vi "STS_IterableDAQ_BK2841.vi"() -> ()   [LabVIEW 2021]
uses:
  <vilib>/express/express analysis/Spectral/Block/exnSpectralBlock spectral measurements RMS poly.vi
  <vilib>/express/express analysis/Spectral/Block/exnSpectralBlock spectral measurements RMS DDT.vi
  <vilib>/express/express analysis/Spectral/XNode/ExpressSpectralMeasurementsBlockNode.xnode
  <vilib>/regexp/Match Regular Expression.xnode
panel:
  in  "Tab Control":enum32{"Page 1", "Page 2"}(tab)
  out "Up Light":bool
  out "Down Light":bool
  out "Acceleration":dynamicdata(graph)
  out "FFT":dynamicdata(graph) caption="Fast Fourier Transform"
  in  "VISA resource name":refnum<visa-resource-name>
  out "BK Measurement":string
  out "Filename Out":path
  in  "Iterations?":i32
  out "Current Iteration":i32
  out "Numeric":dbl
  out "read buffer":string
  out "Resistance":dbl format="%#_6p"
  out "Temp":dbl
  out "Samples / Second":dbl
  out "Resistance Vs Time":dbl(graph)
  in  "Measurement mode":T1(ring)=enum."Resistance and Temp"
  in  "Display State":enum16{"Display ON", "Display OFF"}(ring)=enum."Display OFF"
  in  "Resistance measurement range":T2(ring)
  in  "measurement time":enum16{"FAST", "MED", "SLOW1", "SLOW2"}(ring)
  in  "Measurement speed":enum16{"FAST", "SLOW"}(ring)
  in  "measurement delay time (default 0.003)":dbl=0.003
  out "Array":dbl[](array[numeric])
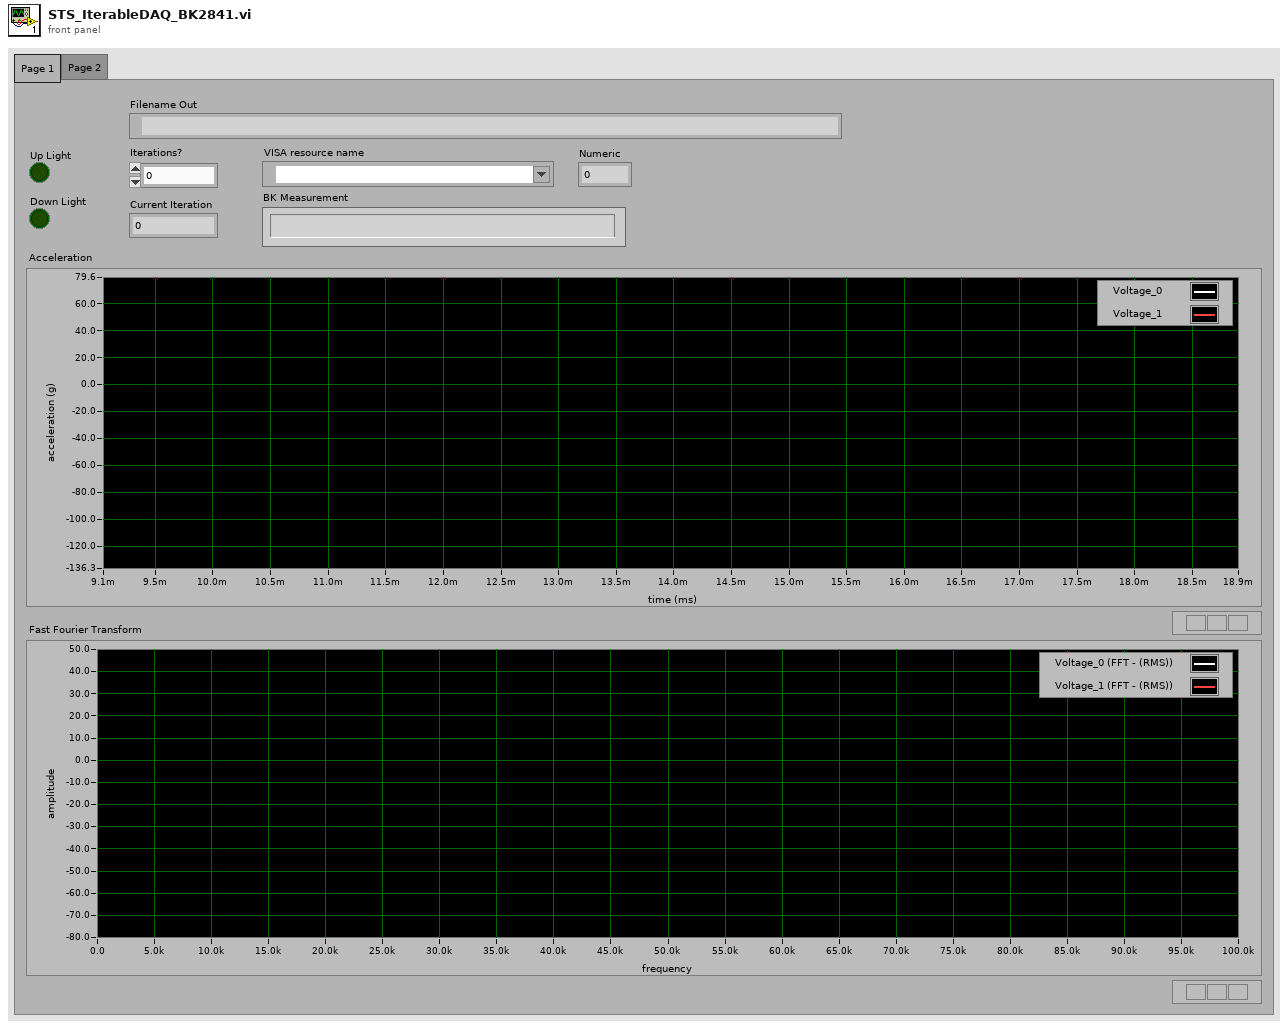
[diagram p1: front panel]
types:
  T1 = enum16{"Resistance", "Resistance and Temp", "Low Power Resistance", "Low Power Resisance and Temp", "Temp"}
  T2 = enum16{"Auto", "20 milli-Ohms", "200 milli-Ohms", "2 Ohms", "20 Ohms", "200 Ohms", "2 k-Ohms", "20 k-Ohms", "100 k-Ohms", "1 M-Ohms", "10 M-Ohms", "100 M-Ohms"}
  T3 = cluster{"averaging mode":u16, "weighting mode":u16, "number of averages":u32}
  T4 = cluster{"dB On (F)":bool, "unwrap phase (F)":bool, "convert to degree (F)":bool}
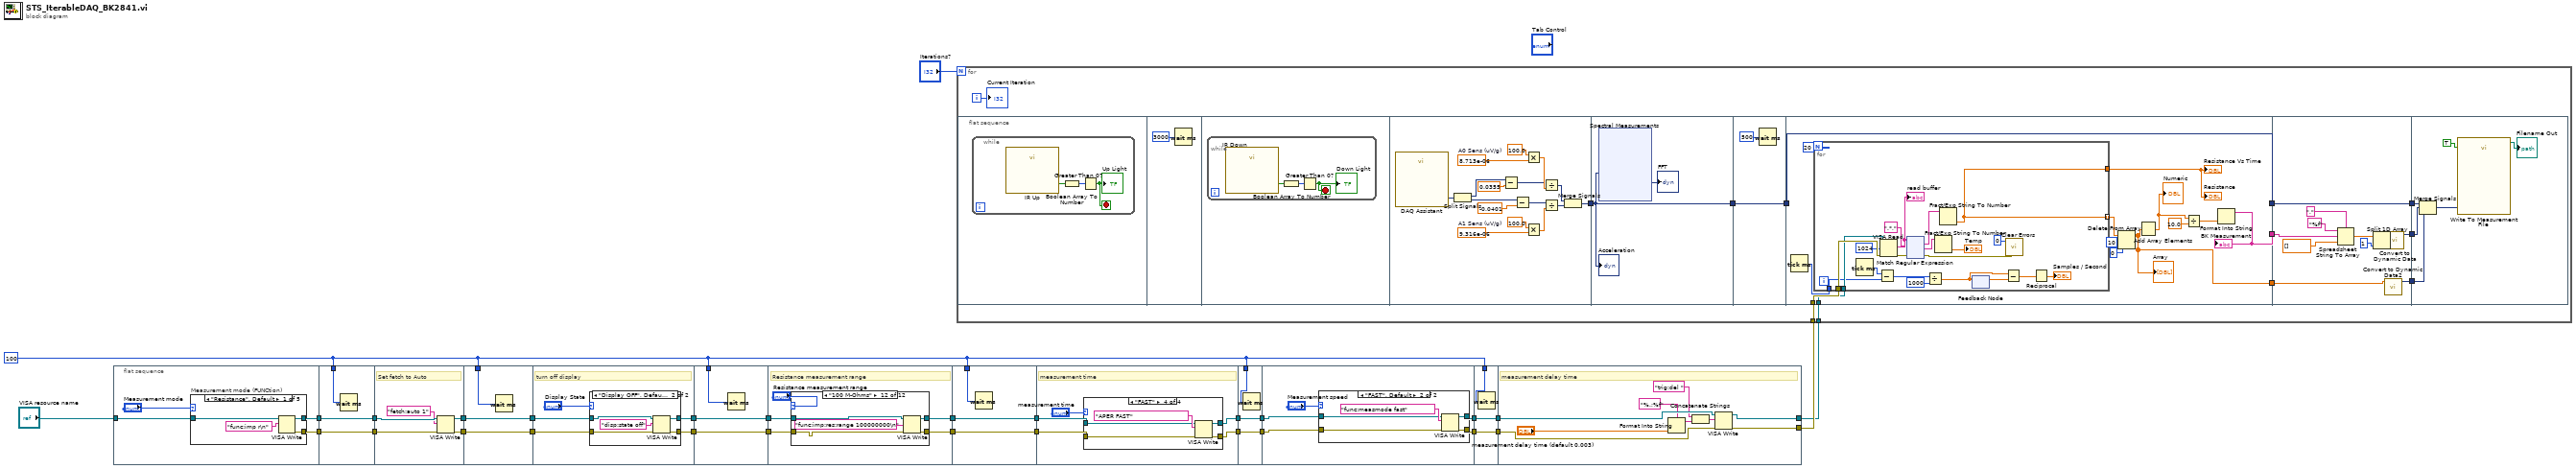
[diagram p0: block diagram]
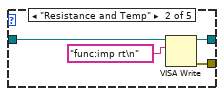
[diagram p2: hidden frame]
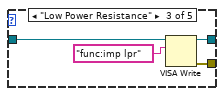
[diagram p3: hidden frame]
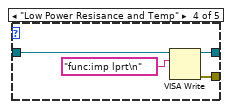
[diagram p4: hidden frame]
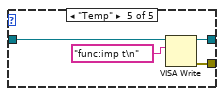
[diagram p5: hidden frame]
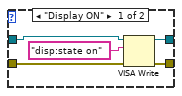
[diagram p6: hidden frame]
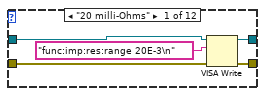
[diagram p7: hidden frame]
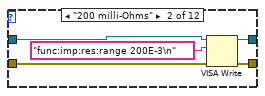
[diagram p8: hidden frame]
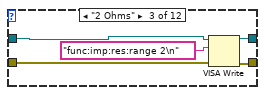
[diagram p9: hidden frame]
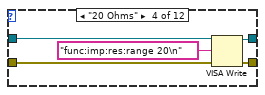
[diagram p10: hidden frame]
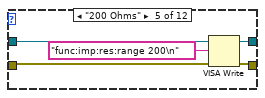
[diagram p11: hidden frame]
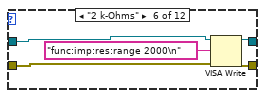
[diagram p12: hidden frame]
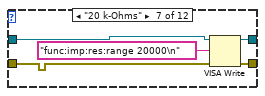
[diagram p13: hidden frame]
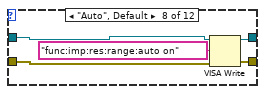
[diagram p14: hidden frame]
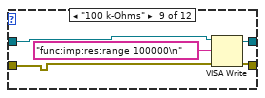
[diagram p15: hidden frame]
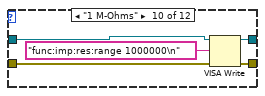
[diagram p16: hidden frame]
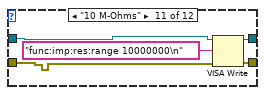
[diagram p17: hidden frame]
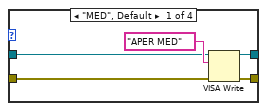
[diagram p18: hidden frame]
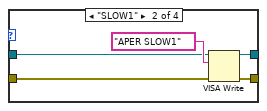
[diagram p19: hidden frame]
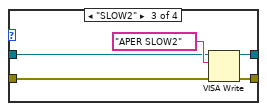
[diagram p20: hidden frame]
diagram:
  w4 = u32 100 ("delay before read (ms)")
  n1 = flat-sequence {
    tunnel: "VISA resource name" -> [w32]
    tunnel: [w30] -> w28
    tunnel: [w31] -> w27
    tunnel: [w56] -> w26
    tunnel: [w55] -> w25
    tunnel: w28 -> [w56]
    tunnel: w27 -> [w55]
    tunnel: w4 -> [w54]
    tunnel: w26 -> [w61]
    tunnel: w25 -> [w60]
    tunnel: [w59] -> w24
    tunnel: [w58] -> w23
    tunnel: w24 -> [w64]
    tunnel: w23 -> [w63]
    tunnel: w4 -> [w62]
    tunnel: [w64] -> w22
    tunnel: [w63] -> w21
    tunnel: w22 -> [w66]
    tunnel: w21 -> [w69]
    tunnel: [w68] -> w20
    tunnel: [w67] -> w19
    tunnel: w20 -> [w81]
    tunnel: w4 -> [w80]
    tunnel: w19 -> [w82]
    tunnel: [w82] -> w18
    tunnel: [w81] -> w17
    tunnel: w18 -> [w85]
    tunnel: w17 -> [w86]
    tunnel: [w83] -> w16
    tunnel: [w84] -> w15
    tunnel: w16 -> [w150]
    tunnel: w15 -> [w149]
    tunnel: [w150] -> w14
    tunnel: [w149] -> w13
    tunnel: w4 -> [w148]
    tunnel: w14 -> [w153]
    tunnel: w13 -> [w154]
    tunnel: [w151] -> w12
    tunnel: [w152] -> w11
    tunnel: w12 -> [w178]
    tunnel: w11 -> [w177]
    tunnel: [w178] -> w10
    tunnel: [w177] -> w9
    tunnel: w4 -> [w176]
    tunnel: w10 -> [w181]
    tunnel: w9 -> [w182]
    tunnel: [w180] -> w8
    tunnel: [w179] -> w7
    tunnel: w8 -> [w196]
    tunnel: w7 -> [w195]
    tunnel: [w196] -> w6
    tunnel: [w195] -> w5
    tunnel: w4 -> [w194]
    tunnel: [w202] -> w1
    tunnel: [w203] -> w2
    tunnel: w6 -> [w204]
    tunnel: w5 -> [w205]
    frame #0 {
      n2 = case "Measurement mode (FUNCtion)" shown="\"Resistance\", Default" "Measurement mode" {
        tunnel: w32 -> [w36 w41 w44 w48 w52]
        tunnel: [w35 w39 w43 w47 w51] -> w31
        tunnel: [w34 w38 w42 w46 w50] -> w30
        frame "Resistance", Default {
          n3 = VISA Write(VISA resource name=w36, write buffer="func:imp r\n") -> (VISA resource name out=w35:refnum<visa-resource-name>, error out=w34:errorcluster)  [unwired: 1 in, 1 out]
        }
        frame "Resistance and Temp" {
          n4 = VISA Write(VISA resource name=w41, write buffer="func:imp rt\n") -> (VISA resource name out=w39:refnum<visa-resource-name>, error out=w38:errorcluster)  [unwired: 1 in, 1 out]
        }
        frame "Low Power Resistance" {
          n5 = VISA Write(VISA resource name=w44, write buffer="func:imp lpr") -> (VISA resource name out=w43:refnum<visa-resource-name>, error out=w42:errorcluster)  [unwired: 1 in, 1 out]
        }
        frame "Low Power Resisance and Temp" {
          n6 = VISA Write(VISA resource name=w48, write buffer="func:imp lprt\n") -> (VISA resource name out=w47:refnum<visa-resource-name>, error out=w46:errorcluster)  [unwired: 1 in, 1 out]
        }
        frame "Temp" {
          n7 = VISA Write(VISA resource name=w52, write buffer="func:imp t\n") -> (VISA resource name out=w51:refnum<visa-resource-name>, error out=w50:errorcluster)  [unwired: 1 in, 1 out]
        }
      }
    }
    frame #1 {
      n8 = Wait (ms)(milliseconds to wait=w54) -> ()  [unwired: 1 out]
    }
    frame #2 {
      # "Set fetch to Auto"
      n9 = VISA Write(VISA resource name=w60, write buffer="fetch:auto 1", error in (no error)=w61) -> (VISA resource name out=w58:refnum<visa-resource-name>, error out=w59:errorcluster)  [unwired: 1 out]
    }
    frame #3 {
      n10 = Wait (ms)(milliseconds to wait=w62) -> ()  [unwired: 1 out]
    }
    frame #4 {
      # "turn off display"
      n11 = case shown="\"Display OFF\", Default" "Display State" {
        tunnel: w69 -> [w70 w78]
        tunnel: [w71 w77] -> w68
        tunnel: [w72 w76] -> w67
        tunnel: w66 -> [w73 w75]
        frame "Display ON" {
          n12 = VISA Write(VISA resource name=w70, write buffer="disp:state on", error in (no error)=w73) -> (VISA resource name out=w71:refnum<visa-resource-name>, error out=w72:errorcluster)  [unwired: 1 out]
        }
        frame "Display OFF", Default {
          n13 = VISA Write(VISA resource name=w78, write buffer="disp:state off", error in (no error)=w75) -> (VISA resource name out=w77:refnum<visa-resource-name>, error out=w76:errorcluster)  [unwired: 1 out]
        }
      }
    }
    frame #5 {
      n14 = Wait (ms)(milliseconds to wait=w80) -> ()  [unwired: 1 out]
    }
    frame #6 {
      # "Resistance measurement range"
      n15 = case shown="\"100 M-Ohms\"" "Resistance measurement range" {
        tunnel: w86 -> [w88 w96 w101 w104 w111 w113 w118 w123 w130 w133 w138 w144]
        tunnel: [w89 w95 w98 w106 w109 w116 w121 w126 w128 w136 w141 w146] -> w84
        tunnel: [w90 w94 w99 w105 w108 w115 w120 w125 w131 w135 w140 w145] -> w83
        tunnel: w85 -> [w91 w93 w100 w103 w110 w114 w119 w124 w129 w134 w139 w143]
        frame "20 milli-Ohms" {
          n16 = VISA Write(VISA resource name=w88, write buffer="func:imp:res:range 20E-3\n", error in (no error)=w91) -> (VISA resource name out=w89:refnum<visa-resource-name>, error out=w90:errorcluster)  [unwired: 1 out]
        }
        frame "200 milli-Ohms" {
          n17 = VISA Write(VISA resource name=w96, write buffer="func:imp:res:range 200E-3\n", error in (no error)=w93) -> (VISA resource name out=w95:refnum<visa-resource-name>, error out=w94:errorcluster)  [unwired: 1 out]
        }
        frame "2 Ohms" {
          n18 = VISA Write(VISA resource name=w101, write buffer="func:imp:res:range 2\n", error in (no error)=w100) -> (VISA resource name out=w98:refnum<visa-resource-name>, error out=w99:errorcluster)  [unwired: 1 out]
        }
        frame "20 Ohms" {
          n19 = VISA Write(VISA resource name=w104, write buffer="func:imp:res:range 20\n", error in (no error)=w103) -> (VISA resource name out=w106:refnum<visa-resource-name>, error out=w105:errorcluster)  [unwired: 1 out]
        }
        frame "200 Ohms" {
          n20 = VISA Write(VISA resource name=w111, write buffer="func:imp:res:range 200\n", error in (no error)=w110) -> (VISA resource name out=w109:refnum<visa-resource-name>, error out=w108:errorcluster)  [unwired: 1 out]
        }
        frame "2 k-Ohms" {
          n21 = VISA Write(VISA resource name=w113, write buffer="func:imp:res:range 2000\n", error in (no error)=w114) -> (VISA resource name out=w116:refnum<visa-resource-name>, error out=w115:errorcluster)  [unwired: 1 out]
        }
        frame "20 k-Ohms" {
          n22 = VISA Write(VISA resource name=w118, write buffer="func:imp:res:range 20000\n", error in (no error)=w119) -> (VISA resource name out=w121:refnum<visa-resource-name>, error out=w120:errorcluster)  [unwired: 1 out]
        }
        frame "Auto", Default {
          n23 = VISA Write(VISA resource name=w123, write buffer="func:imp:res:range:auto on", error in (no error)=w124) -> (VISA resource name out=w126:refnum<visa-resource-name>, error out=w125:errorcluster)  [unwired: 1 out]
        }
        frame "100 k-Ohms" {
          n24 = VISA Write(VISA resource name=w130, write buffer="func:imp:res:range 100000\n", error in (no error)=w129) -> (VISA resource name out=w128:refnum<visa-resource-name>, error out=w131:errorcluster)  [unwired: 1 out]
        }
        frame "1 M-Ohms" {
          n25 = VISA Write(VISA resource name=w133, write buffer="func:imp:res:range 1000000\n", error in (no error)=w134) -> (VISA resource name out=w136:refnum<visa-resource-name>, error out=w135:errorcluster)  [unwired: 1 out]
        }
        frame "10 M-Ohms" {
          n26 = VISA Write(VISA resource name=w138, write buffer="func:imp:res:range 10000000\n", error in (no error)=w139) -> (VISA resource name out=w141:refnum<visa-resource-name>, error out=w140:errorcluster)  [unwired: 1 out]
        }
        frame "100 M-Ohms" {
          n27 = VISA Write(VISA resource name=w144, write buffer="func:imp:res:range 100000000\n", error in (no error)=w143) -> (VISA resource name out=w146:refnum<visa-resource-name>, error out=w145:errorcluster)  [unwired: 1 out]
        }
      }
    }
    frame #7 {
      n28 = Wait (ms)(milliseconds to wait=w148) -> ()  [unwired: 1 out]
    }
    frame #8 {
      # "measurement time"
      n29 = case shown="\"FAST\"" "measurement time" {
        tunnel: w154 -> [w156 w164 w169 w171]
        tunnel: [w157 w163 w166 w174] -> w152
        tunnel: [w158 w162 w167 w173] -> w151
        tunnel: w153 -> [w159 w161 w168 w172]
        frame "MED", Default {
          n30 = VISA Write(VISA resource name=w156, write buffer="APER MED", error in (no error)=w159) -> (VISA resource name out=w157:refnum<visa-resource-name>, error out=w158:errorcluster)  [unwired: 1 out]
        }
        frame "SLOW1" {
          n31 = VISA Write(VISA resource name=w164, write buffer="APER SLOW1", error in (no error)=w161) -> (VISA resource name out=w163:refnum<visa-resource-name>, error out=w162:errorcluster)  [unwired: 1 out]
        }
        frame "SLOW2" {
          n32 = VISA Write(VISA resource name=w169, write buffer="APER SLOW2", error in (no error)=w168) -> (VISA resource name out=w166:refnum<visa-resource-name>, error out=w167:errorcluster)  [unwired: 1 out]
        }
        frame "FAST" {
          n33 = VISA Write(VISA resource name=w171, write buffer="APER FAST", error in (no error)=w172) -> (VISA resource name out=w174:refnum<visa-resource-name>, error out=w173:errorcluster)  [unwired: 1 out]
        }
      }
    }
    frame #9 {
      n34 = Wait (ms)(milliseconds to wait=w176) -> ()  [unwired: 1 out]
    }
    frame #10 {
      n35 = case shown="\"FAST\", Default" "Measurement speed" {
        tunnel: w182 -> [w187 w189]
        tunnel: [w186 w192] -> w179
        tunnel: [w185 w191] -> w180
        tunnel: w181 -> [w184 w190]
        frame "SLOW" {
          n36 = VISA Write(VISA resource name=w187, write buffer="func:measmode slow", error in (no error)=w184) -> (VISA resource name out=w186:refnum<visa-resource-name>, error out=w185:errorcluster)  [unwired: 1 out]
        }
        frame "FAST", Default {
          n37 = VISA Write(VISA resource name=w189, write buffer="func:measmode fast", error in (no error)=w190) -> (VISA resource name out=w192:refnum<visa-resource-name>, error out=w191:errorcluster)  [unwired: 1 out]
        }
      }
    }
    frame #11 {
      n38 = Wait (ms)(milliseconds to wait=w194) -> ()  [unwired: 1 out]
    }
    frame #12 {
      # "measurement delay time"
      n39 = Format Into String(format string="%.;%f", "measurement delay time (default 0.003)") -> (resulting string=w198:string)  [unwired: 2 in, 1 out]
      n40 = Concatenate Strings("trig:del " ("write buffer"), w198) -> (w197:string)
      n41 = VISA Write(VISA resource name=w205, write buffer=w197, error in (no error)=w204) -> (VISA resource name out=w202:refnum<visa-resource-name>, error out=w203:errorcluster)  [unwired: 1 out]
    }
  }
  n42 = for {
    N: "Iterations?" -> [_]
    tunnel: w2 -> [w209]
    tunnel: w1 -> [w208]
    i -> [w210]
    n43 = flat-sequence {
      tunnel: [w238] -> w217
      tunnel: w217 -> [w241]
      tunnel: [w241] -> w216
      tunnel: w216 -> [w253]
      tunnel: [w253] -> w215
      tunnel: [w265] -> w214
      tunnel: w215 -> [w268]
      tunnel: [w268] -> w213
      tunnel: w209 -> [w267]
      tunnel: w208 -> [w266]
      tunnel: [w255] -> w206
      tunnel: w214 -> [w408]
      tunnel: w213 -> [w409]
      tunnel: [w410] -> w212
      tunnel: [w409] -> w211
      tunnel: [w407] -> w207
      tunnel: w206 -> [w406]
      tunnel: w212 -> [w421]
      tunnel: w211 -> [w422]
      tunnel: w207 -> [w417]
      frame #0 {
        n44 = while {
          stop <- w219 stop-if-true
          n45 = call "IR Up"() -> ("data"=w218:bool[])  [unwired: 17 in, 2 out]
          n46 = Boolean Array To Number(Boolean array=w218) -> (number=w220:u32)
          n47 = Greater Than 0?(x=w220) -> (x > 0?=w219:bool)
          "Up Light" <- w219
        }
      }
      frame #1 {
        n48 = Wait (ms)(milliseconds to wait=u32 3000) -> ()  [unwired: 1 out]
      }
      frame #2 {
        n49 = while {
          stop <- w223 stop-if-true
          n50 = call "IR Down"() -> ("data"=w222:bool[])  [unwired: 17 in, 2 out]
          n51 = Boolean Array To Number(Boolean array=w222) -> (number=w224:u32)
          n52 = Greater Than 0?(x=w224) -> (x > 0?=w223:bool)
          "Down Light" <- w223
        }
      }
      frame #3 {
        w232 = 8.713e-06  # A0 Sens (uV/g)
        w228 = 9.316e-06  # A1 Sens (uV/g)
        n53 = call "DAQ Assistant"() -> ("data"=w237:dynamicdata)  [unwired: 17 in, 2 out]
        n54 = Split Signals(w237) -> (w235:dynamicdata, w236:dynamicdata)  [unwired: 2 in]
        n55 = Subtract(x=w235, y=0.0355) -> (x-y=w230:dynamicdata)
        n56 = Subtract(x=w236, y=-0.0401) -> (x-y=w226:dynamicdata)
        n57 = Multiply(x=100.0, y=w232) -> (x*y=w231:dbl)
        n58 = Multiply(x=100.0, y=w228) -> (x*y=w227:dbl)
        n59 = Divide(x=w230, y=w231) -> (x/y=w229:dynamicdata)
        n60 = Divide(x=w226, y=w227) -> (x/y=w225:dynamicdata)
        n61 = Merge Signals(w229, w225) -> (w238:dynamicdata)
      }
      frame #4 {
        n62 = xnode "Spectral Measurements"("Signals"=w241) -> ("FFT - (RMS)"=→"FFT":dynamicdata)  [unwired: 1 in, 2 out]
        "Acceleration" <- w241
      }
      frame #5 {
        n63 = Wait (ms)(milliseconds to wait=u32 500 ("delay before read (ms)")) -> ()  [unwired: 1 out]
      }
      frame #6 {
        n64 = Tick Count (ms)() -> (millisecond timer value=w264:u32)
        n65 = for {
          N: 20 -> [_]
          tunnel: w267 -> [w275]
          tunnel: w266 -> [w273]
          tunnel: w264 -> [w272]
          tunnel: [w271] -> w260
          tunnel: [w271] -> w258 mode=indexing
          n66 = Tick Count (ms)() -> (millisecond timer value=w282:u32)
          n67 = Subtract(x=w282, y=w272) -> (x-y=w284:u32)
          n68 = VISA Read(VISA resource name=w273, byte count=u32 1024, error in (no error)=w275) -> (read buffer=w281:string, error out=w280:errorcluster)  [unwired: 2 out]
          "read buffer" <- w281
          n69 = xnode "Match Regular Expression"("input string"=w281, "regular expression"=".*,", "error in"=w280) -> ("whole match"=w278:string, "after match"=w279:string, "error out"=w270:errorcluster)  [unwired: 3 in, 2 out]
          n70 = Divide(x=w284, y=u32 1000) -> (x/y=w285:dbl)
          n71 = Fract/Exp String To Number(string=w279) -> (number=→"Temp":dbl)  [unwired: 3 in, 1 out]
          n72 = Fract/Exp String To Number(string=w278) -> (number=w271:dbl)  [unwired: 3 in, 1 out]
          n73 = feedback #1() -> (w286:dbl)  [unwired: 1 in]
          n74 = feedback-in #1(w285) -> ()
          n75 = Subtract(x=w285, y=w286) -> (x-y=w287:dbl)
          n76 = call <vilib>:"Clear Errors.vi"("error in (no error)"=w270, "specific error code to clear (0: all)"=0) -> ()  [unwired: 4 in, 2 out]
          n77 = Reciprocal(x=w287) -> (1/x=→"Samples / Second":dbl)
        }
        "Resistance" <- w260
        "Resistance Vs Time" <- w260
        n78 = Delete From Array(array=w258, length=10, index=0) -> (array with subset deleted=w255:dbl[])  [unwired: 1 out]
        "Array" <- w255
        n79 = Add Array Elements(numeric array=w255) -> (sum=w259:dbl)
        "Numeric" <- w259
        n80 = Divide(x=w259, y=10.0) -> (x/y=w261:dbl)
        n81 = Format Into String(w261) -> (resulting string=w265:string)  [unwired: 3 in, 1 out]
        "BK Measurement" <- w265
      }
      frame #7 {
        n82 = Spreadsheet String To Array(delimiter (Tab)=",", format string="%f", spreadsheet string=w408, array type (2D Dbl)=dbl[] []) -> (array=w415:dbl[])
        n83 = Split 1D Array(array=w415, index=1) -> (first subarray=w416:dbl[])  [unwired: 1 out]
        n84 = call "Convert to Dynamic Data2"("Array"=w406) -> ("Dynamic Data Type"=w407:dynamicdata)  [unwired: 3 in]
        n85 = call "Convert to Dynamic Data"("Array"=w416) -> ("Dynamic Data Type"=w410:dynamicdata)  [unwired: 3 in]
      }
      frame #8 {
        n86 = Merge Signals(w422, w421, w417) -> (w420:dynamicdata)
        n87 = call "Write To Measurement File"("Signals"=w420, "Reset"=TRUE) -> ("Filename Out"=→"Filename Out":path)  [unwired: 15 in, 2 out]
      }
    }
    "Current Iteration" <- w210
  }
